vi "Estimate All Positions - Star Configuration.vi"(8 "Input AnchorArray":refnum<class "Anchor.lvclass">[](array[class]), 11 "Tag.lvclass":refnum<class "Tag.lvclass">) -> (0 "Output AnchorArray":refnum<class "Anchor.lvclass">[](array[class]), 2 "Intersections":T1(array[cluster]), 3 "PositionCluster [tagID, x, y, anchorID, distances]":T2)   [LabVIEW 2014, in "Position.lvclass"]
doc: "This VI estimates the Tag's (x,y)-coordinates based on the input array of Anchors. For a swarm implementation (see system documentation) TagDistanceArray should be given too."
uses:
  Position.lvclass
  Anchor/Anchor.lvclass
  Tag.lvclass
panel:
  out "error out":errorcluster
  in  "error in (no error)":errorcluster
  out "TagID":dbl
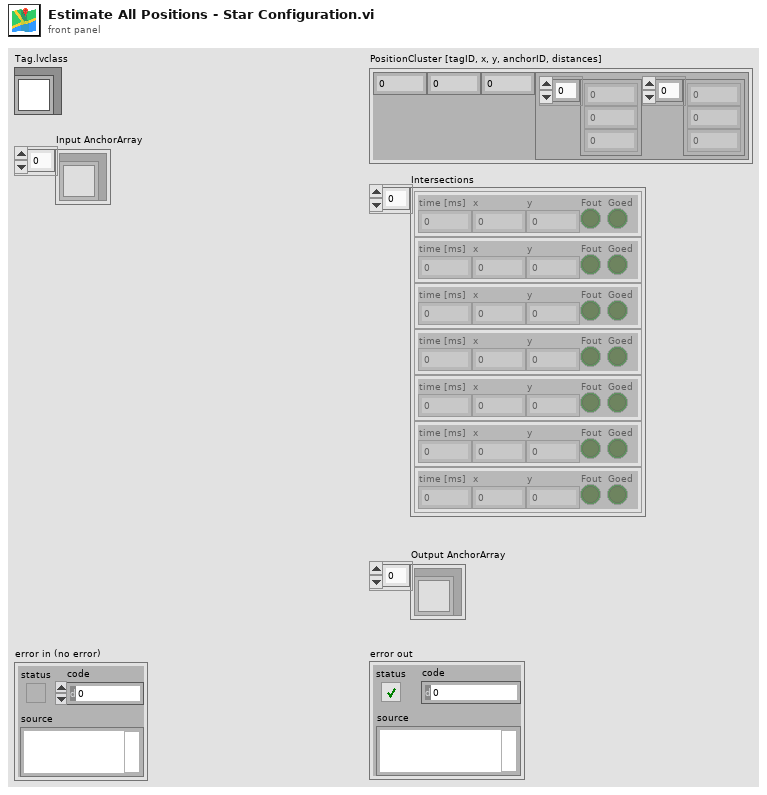
[diagram p1: front panel]
types:
  T1 = cluster{"time [ms]":dbl, "x":dbl, "y":dbl, "Fout":bool, "Goed":bool}[]
  T2 = cluster{"tagID":dbl, "X":dbl, "Y":dbl, "anchorIDDistanceCluster":cluster{"anchorIDArray":dbl[], "anchorDistanceArray":dbl[]}}
  T3 = cluster{"time [ms]":dbl, "y":dbl, "x":dbl, "Fout":bool, "Goed":bool}[]
  T4 = cluster{"anchorIDArray":dbl[], "anchorDistanceArray":dbl[]}
  T5 = cluster{"Tag.lvclass":refnum<class "Tag.lvclass">, "Distance":dbl}[]
  T6 = cluster{"Time [ms]":dbl, "x":dbl, "y":dbl, "Fout":bool, "Goed":bool}[]
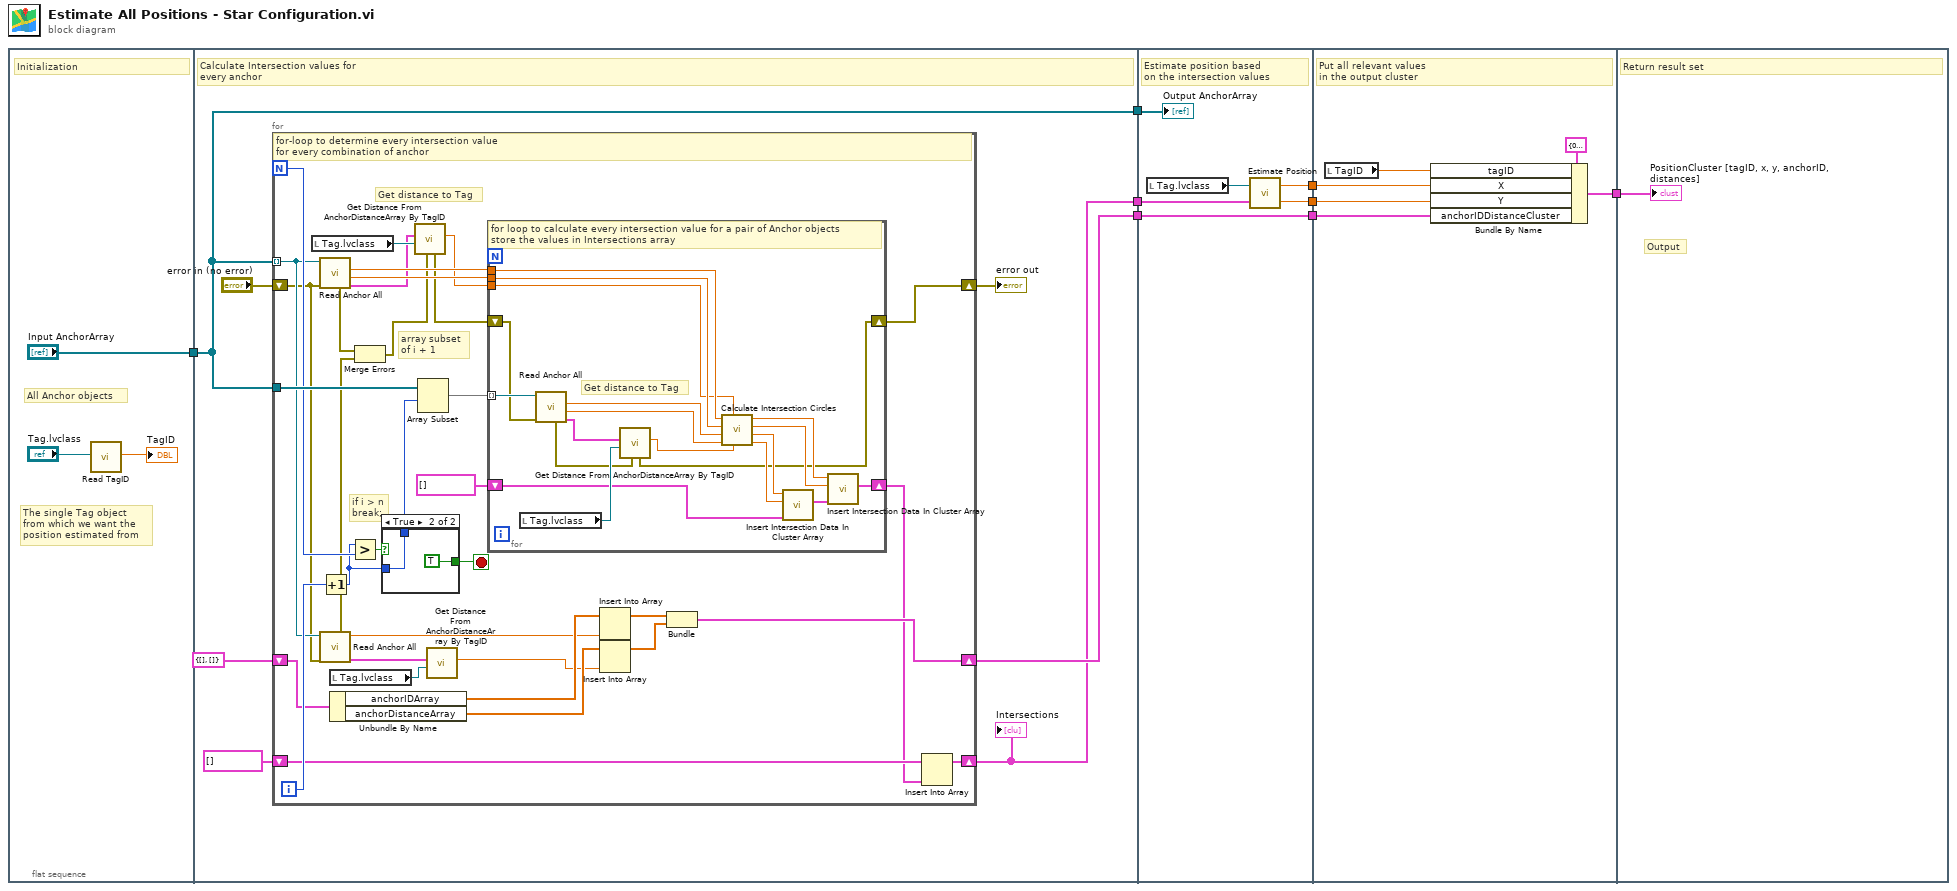
[diagram p0: block diagram]
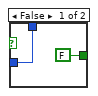
[diagram p2: hidden frame]
diagram:
  n1 = flat-sequence {
    tunnel: ["Input AnchorArray"] -> w8
    tunnel: w8 -> [w14]
    tunnel: [w17] -> w3
    tunnel: [w15] -> w2
    tunnel: [w14] -> w1
    tunnel: [w81] -> w7
    tunnel: [w80] -> w6
    tunnel: [w79] -> w4
    tunnel: w3 -> [w79]
    tunnel: w2 -> [w78]
    tunnel: w1 -> [w77]
    tunnel: w7 -> [w85]
    tunnel: w6 -> [w84]
    tunnel: [w83] -> w5
    tunnel: w4 -> [w82]
    tunnel: w5 -> [w88]
    frame #0 {
      # "The single Tag object\nfrom which we want the \nposition estimated from"
      # "All Anchor objects"
      # "Initialization"
      n2 = call "Read TagID.vi"("Tag in"="Tag.lvclass") -> ("TagID"=→"TagID":dbl)  [unwired: 16 in, 2 out]
    }
    frame #1 {
      # "Calculate Intersection values for \nevery anchor"
      n3 = for {
        N -> [w44]
        tunnel: w14 -> [w51]
        tunnel: w14 -> [w39] mode=indexing
        shift-right: [w29] -> w17
        shift-left: T4 {"anchorIDArray"=[], "anchorDistanceArray"=[]} ("anchorIDDistanceCluster") -> [w36]
        shift-right: [w27] -> w15
        shift-left: T3 [] ("Intersections 2") -> [w28]
        shift-right: [w24] -> w12
        shift-left: "error in (no error)" -> [w19]
        i -> [w48]
        stop <- w42 stop-if-true
        # "array subset\nof i + 1"
        # "if i > n\nbreak;"
        # "Get distance to Tag"
        # "for-loop to determine every intersection value\nfor every combination of anchor"
        n4 = local read "Tag.lvclass"() -> (w47:refnum<class "Tag.lvclass">)
        n5 = call "Read Anchor All.vi"("error in (no error)"=w19, "Anchor in"=w39) -> ("TagDistanceArray"=w46:T5, "AnchorY"=w49:dbl, "AnchorX"=w50:dbl, "error out"=w22:errorcluster)  [unwired: 4 in, 2 out]
        n6 = call "Read Anchor All.vi"("error in (no error)"=w19, "Anchor in"=w39) -> ("TagDistanceArray"=w38:T5, "AnchorID"=w33:dbl, "error out"=w23:errorcluster)  [unwired: 4 in, 3 out]
        n7 = Increment(x=w48) -> (x+1=w41:i32)
        n8 = local read "Tag.lvclass"() -> (w37:refnum<class "Tag.lvclass">)
        n9 = Unbundle By Name(w36) -> ("anchorIDArray"=w35:dbl[], "anchorDistanceArray"=w34:dbl[])
        n10 = Greater?(x=w41, y=w44) -> (0:w43:bool)
        n11 = Merge Errors(w22, w23) -> (w21:errorcluster)
        n12 = case shown="True" w43 {
          tunnel: [FALSE TRUE] -> w42
          tunnel: w41 -> [w53 w55]
          tunnel: [w53 w55] -> w40
          frame False {
          }
          frame True {
          }
        }
        n13 = call "Get Distance From AnchorDistanceArray By TagID.vi"("error in (no error)"=w21, "Tag.lvclass"=w47, "Input TagDistanceArray"=w46) -> ("Distance"=w45:dbl, "error out"=w20:errorcluster)  [unwired: 7 in]
        n14 = Array Subset(array=w51, index=w40) -> (w25:refnum<class "Anchor.lvclass">[])  [unwired: 1 in]
        n15 = call "Get Distance From AnchorDistanceArray By TagID.vi"("Tag.lvclass"=w37, "Input TagDistanceArray"=w38) -> ("Distance"=w32:dbl)  [unwired: 8 in, 1 out]
        n16 = for {
          shift-right: [w62] -> w26
          shift-left: T1 [] ("Intersections 2") -> [w66]
          tunnel: w25 -> [w75] mode=indexing
          tunnel: w50 -> [w74]
          tunnel: w49 -> [w73]
          tunnel: w45 -> [w70]
          shift-right: [w57] -> w24
          shift-left: w20 -> [w59]
          # "Get distance to Tag"
          # "for loop to calculate every intersection value for a pair of Anchor objects\nstore the values in Intersections array"
          n17 = local read "Tag.lvclass"() -> (w72:refnum<class "Tag.lvclass">)
          n18 = call "Read Anchor All.vi"("error in (no error)"=w59, "Anchor in"=w75) -> ("TagDistanceArray"=w69:T5, "AnchorY"=w67:dbl, "AnchorX"=w68:dbl, "error out"=w58:errorcluster)  [unwired: 4 in, 2 out]
          n19 = call "Get Distance From AnchorDistanceArray By TagID.vi"("error in (no error)"=w58, "Tag.lvclass"=w72, "Input TagDistanceArray"=w69) -> ("Distance"=w71:dbl, "error out"=w57:errorcluster)  [unwired: 7 in]
          n20 = call "Calculate Intersection Circles.vi"("r2"=w71, "r1"=w70, "d"=w67, "c"=w68, "b"=w73, "a"=w74) -> ("y2"=w65:dbl, "x2"=w64:dbl, "y1"=w60:dbl, "x1"=w61:dbl)  [unwired: 2 in]
          n21 = call "Insert Intersection Data In Cluster Array.vi"("ClusterArray"=w66, "Y"=w65, "X"=w64) -> ("Intersections"=w63:T6)  [unwired: 8 in]
          n22 = call "Insert Intersection Data In Cluster Array.vi"("ClusterArray"=w63, "Y"=w60, "X"=w61) -> ("Intersections"=w62:T6)  [unwired: 8 in]
        }
        n23 = Insert Into Array(array=w35, new element=w33) -> (w31:dbl[])  [unwired: 1 in]
        n24 = Insert Into Array(array=w34, new element=w32) -> (w30:dbl[])  [unwired: 1 in]
        n25 = Bundle("anchorIDArray"=w31, "anchorDistanceArray"=w30) -> (w29:T4)  [unwired: 1 in]
        n26 = Insert Into Array(array=w28, new element=w26) -> (w27:T3)  [unwired: 1 in]
      }
      "Intersections" <- w15
      "error out" <- w12
    }
    frame #2 {
      # "Estimate position based\non the intersection values"
      n27 = local read "Tag.lvclass"() -> (w76:refnum<class "Tag.lvclass">)
      n28 = call "Estimate Position.vi"("Intersections"=w78, "Tag.lvclass"=w76) -> ("Y"=w80:dbl, "X"=w81:dbl)
      "Output AnchorArray" <- w77
    }
    frame #3 {
      # "Put all relevant values\nin the output cluster"
      n29 = local read "TagID"() -> (w86:dbl)
      n30 = Bundle By Name(cluster=T2 {"tagID"=0.0, "X"=0.0, "Y"=0.0, "anchorIDDistanceCluster"={"anchorIDArray"=[], "anchorDistanceArray"=[]}} ("PositionCluster [tagID, x, y, anchorID, distances] 2"), "tagID"=w86, "X"=w85, "Y"=w84, "anchorIDDistanceCluster"=w82) -> (w83:T2)
    }
    frame #4 {
      # "Output"
      # "Return result set"
      "PositionCluster [tagID, x, y, anchorID, distances]" <- w88
    }
  }
